vi "Prepare metrics.vi"(1 "LOG Gas":bool, 2 "LO G RF":bool) -> (0 "Metrics":cluster{string, "O2":dbl}[](array[cluster]))   [LabVIEW 2023]
uses:
  global variables.vi
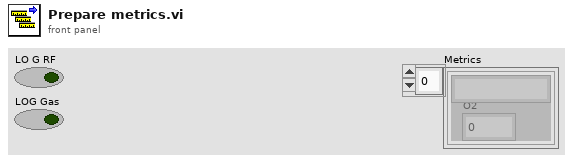
[diagram p1: front panel]
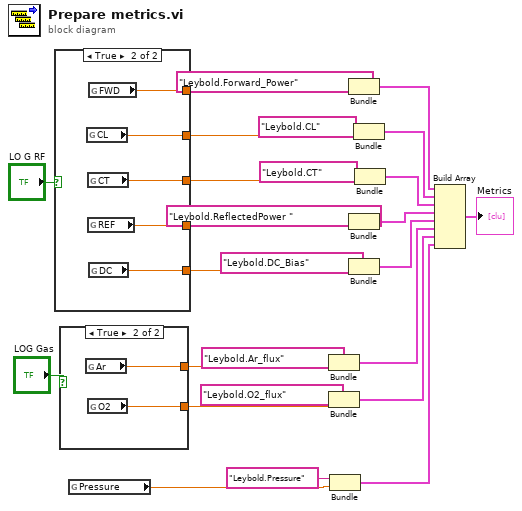
[diagram p0: block diagram]
diagram:
  n1 = case shown="True" "LO G RF" {
    tunnel: [_ w32] -> w19
    tunnel: [_ w31] -> w18
    tunnel: [_ w30] -> w15
    tunnel: [_ w29] -> w14
    tunnel: [_ w28] -> w11
    frame False {
    }
    frame True {
      n2 = global read "global variables.vi" "CL"() -> (w31:dbl)
      n3 = global read "global variables.vi" "CT"() -> (w30:dbl)
      n4 = global read "global variables.vi" "REF"() -> (w29:dbl)
      n5 = global read "global variables.vi" "FWD"() -> (w32:dbl)
      n6 = global read "global variables.vi" "DC"() -> (w28:dbl)
    }
  }
  n7 = case shown="True" "LOG Gas" {
    tunnel: [_ w34] -> w10
    tunnel: [_ w33] -> w7
    frame False {
    }
    frame True {
      n8 = global read "global variables.vi" "Ar"() -> (w34:dbl)
      n9 = global read "global variables.vi" "O2"() -> (w33:dbl)
    }
  }
  n10 = global read "global variables.vi" "Pressure"() -> (w3:dbl)
  n11 = Bundle("Leybold.Ar_flux", "Ar"=w10) -> (w22:cluster{string, "Ar":dbl})  [unwired: 1 in]
  n12 = Bundle("Leybold.O2_flux", "O2"=w7) -> (w21:cluster{string, "O2":dbl})  [unwired: 1 in]
  n13 = Bundle("Leybold.Pressure", "Pressure"=w3) -> (w1:cluster{string, "Pressure":dbl})  [unwired: 1 in]
  n14 = Bundle("Leybold.Forward_Power", "FWD"=w19) -> (w27:cluster{string, "FWD":dbl})  [unwired: 1 in]
  n15 = Bundle("Leybold.ReflectedPower ", "REF"=w14) -> (w24:cluster{string, "REF":dbl})  [unwired: 1 in]
  n16 = Bundle("Leybold.DC_Bias", "DC"=w11) -> (w23:cluster{string, "DC":dbl})  [unwired: 1 in]
  n17 = Bundle("Leybold.CL", "CL"=w18) -> (w26:cluster{string, "CL":dbl})  [unwired: 1 in]
  n18 = Bundle("Leybold.CT", "CT"=w15) -> (w25:cluster{string, "CT":dbl})  [unwired: 1 in]
  n19 = Build Array(w27, w26, w25, w24, w23, w22, w21, w1) -> (→"Metrics":cluster{string, "Pressure":dbl}[])
